vi "TDToVariant.vi"(2 "error in (no error)":errorcluster={"status"=FALSE, "code"=1097, "source"="Call Library Function Node in TDToVariant.vi->LVH5TGetLVType.vi:1->H5Dread (Variant).vi->Simple H5Dread (Variant).vi->TestPQsAndBools.vi"}, 3 "Type Descriptor":i16[](array[numeric]) format="%.0x") -> (0 "error out":errorcluster, 1 "Default Data":variant)   [LabVIEW 2017]
panel:
  out "*(type *) &x":string
  in  "dummy control":variant
  # "LVHDF5 Toolkit\nCopyright (c) 2005-2013 by Jason D. Sommerville\nCopyright (c) 2014 by UPVI, LLC.\n\nThis use and distribution of this file is governed by the terms found in \nLICENSE.txt distributed with this toolkit and installed at\n <user.lib>\\_lvhdf5\\LICENSE.txt"
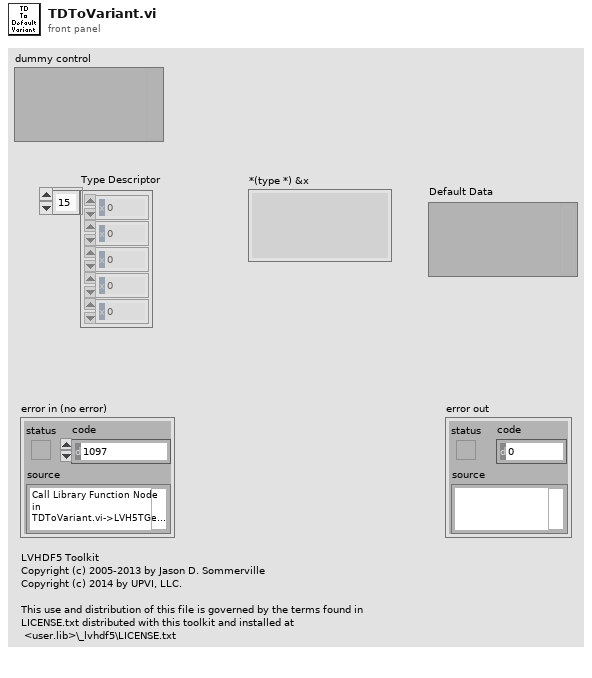
[diagram p1: front panel]
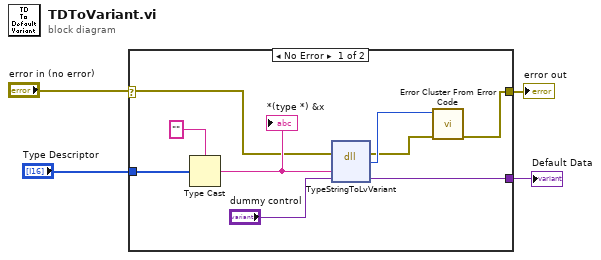
[diagram p0: block diagram]
diagram:
  n1 = case shown="No Error" "error in (no error)" {
    selector: "error in (no error)" -> [w7 w14]
    tunnel: "Type Descriptor" -> [w13 _]
    tunnel: [w11 _] -> w3
    tunnel: [w8 w14] -> w2
    frame No Error {
      n2 = Type Cast(type="", x=w13) -> (*(type *) &x=w12:string)
      "*(type *) &x" <- w12
      n3 = dll-call lib="LabVIEW" fn="TypeStringToLvVariant"(error in=w7, "td"=w12, "plvvar"="dummy control") -> (error out=w9:errorcluster, "return type"=w10:i32, "plvvar"=w11:variant)  [unwired: 3 in, 1 out]
      n4 = call <vilib>:"Error Cluster From Error Code.vi"("error in (no error)"=w9, "error code (0)"=w10) -> ("error out"=w8:errorcluster)  [unwired: 7 in]
    }
    frame Error {
    }
  }
  "Default Data" <- w3
  "error out" <- w2
